vi "SingleComplex (Scalar) to String.vi"(7 "Use System Default Notation (F)":bool, 11 "Value (CSG)":csg) -> (3 "Value (String)":string)   [LabVIEW 2013, in "OpenScalar.lvlib"]
uses:
  OpenScalar.lvlib
  FinalStringFormatting.vi
  Get Decimal Separator.vi
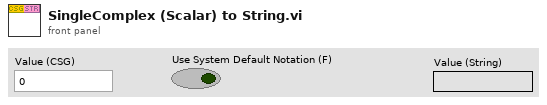
[diagram p1: front panel]
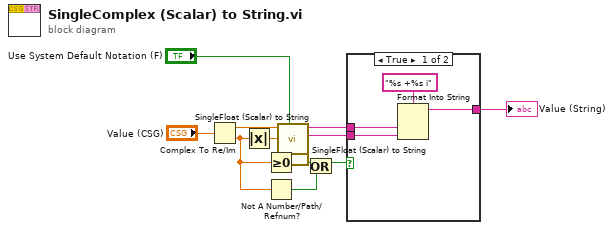
[diagram p0: block diagram]
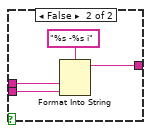
[diagram p2: hidden frame]
diagram:
  n1 = Complex To Re/Im(x + iy="Value (CSG)") -> (x=w10:sgl, y=w2:sgl)
  n2 = Absolute Value(x=w2) -> (abs(x)=w5:sgl)
  n3 = Greater Or Equal To 0?(x=w2) -> (x >= 0?=w4:bool)
  n4 = Not A Number/Path/Refnum?(number/path/refnum=w2) -> (NaN/Path/Refnum?=w1:bool)
  n5 = call "SingleFloat (Scalar) to String.vi"("Use System Default Notation (F)"="Use System Default Notation (F)", "Value (Single)"=w10) -> ("Value (String)"=w8:string)  [unwired: 9 in]
  n6 = call "SingleFloat (Scalar) to String.vi"("Use System Default Notation (F)"="Use System Default Notation (F)", "Value (Single)"=w5) -> ("Value (String)"=w7:string)  [unwired: 9 in]
  n7 = Or(x=w4, y=w1) -> (x .or. y?=w3:bool)
  n8 = case shown="True" w3 {
    tunnel: w8 -> [w15 w19]
    tunnel: w7 -> [w13 w17]
    tunnel: [w12 w16] -> w6
    frame True {
      n9 = Format Into String(format string="%s +%s i", w15, w13) -> (resulting string=w12:string)  [unwired: 2 in, 1 out]
    }
    frame False {
      n10 = Format Into String(format string="%s -%s i", w19, w17) -> (resulting string=w16:string)  [unwired: 2 in, 1 out]
    }
  }
  "Value (String)" <- w6
